vi "Init_Test.vi"(8 "error in (no error)":errorcluster caption="entrée d'erreur (pas d'erreur)", 11 "Get_Voltage en entrée":refnum<class "Start_Continuous_Ana.lvclass">) -> (0 "error out":errorcluster caption="sortie d'erreur", 3 "Get_Voltage en sortie":refnum<class "Start_Continuous_Ana.lvclass">)   [LabVIEW 2020, in "Library Test.lvlib" / "Start_Continuous_Ana.lvclass"]
uses:
  Start_Continuous_Ana.lvclass
  C:/Users/ngarcin/OneDrive - Altyor/Standard TB/Suite TB45/Class/Test/Test (Default)/Test (Default).lvclass
  Commun VI/TypeDef/Commande Test/Commande Value Type.ctl
  Commun VI/TypeDef/Commande Test/Commande Type Test.ctl
  Commun VI/TypeDef/Variable Printable.ctl
  Test_Wtih_Instr/Test_With_Inst.lvclass
  Instrument/Instrument (Default)/Class Instrument (Default).lvclass
  Commun VI/Library Commun.lvlib
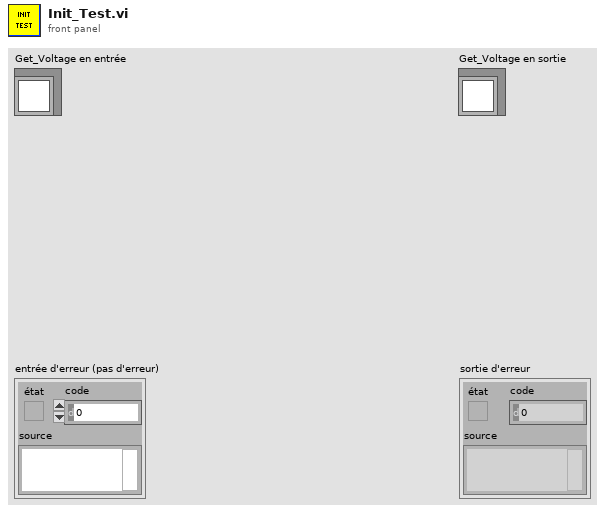
[diagram p1: front panel]
types:
  T1 = typedef "Variable Printable.ctl" = string
  T2 = enum16{"Get Variable", "Get All Variables", "Set Variable", "Delete Variable", "Delete All Variable"}
  T3 = typedef "Library Commun.lvlib/Commande Type Test.ctl" = enum16{"Function", "Test", "Calculation"}
  T4 = typedef "Library Commun.lvlib/Commande Value Type.ctl" = enum16{"None", "String", "Number", "Timestamp", "Boolean", "Array"}
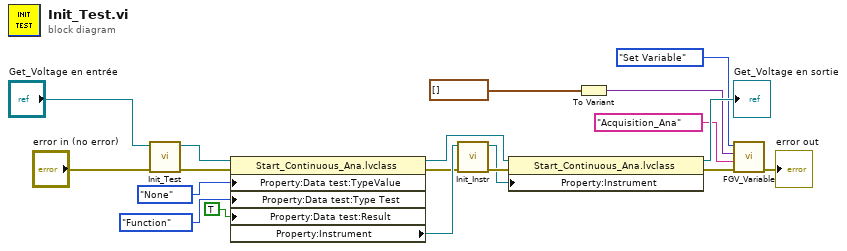
[diagram p0: block diagram]
diagram:
  n1 = call-parent "Init_Test.vi"("error in (no error)"="error in (no error)", "Test_With_Inst en entrée"="Get_Voltage en entrée") -> ("error out"=w16:errorcluster, "Test_With_Inst en sortie"=w17:refnum<class "Start_Continuous_Ana.lvclass">)  [unwired: 8 in]
  n2 = property class="Start_Continuous_Ana.lvclass"(reference=w17, error in=w16, "Property:Data test:TypeValue"=Commande_Value_Type."None" ("TypeValue"), "Property:Data test:Type Test"=Commande_Type_Test."Function" ("Type Test"), "Property:Data test:Result"=TRUE ("Result")) -> (reference out=w11:refnum<class "Start_Continuous_Ana.lvclass">, error out=w1:errorcluster, "Property:Instrument"=w2:refnum<class "Class Instrument (Default).lvclass">)
  n3 = call-dynamic "Init_Instr.vi"("error in (no error)"=w1, "Class Instrument (Default) en entrée"=w2) -> ("error out"=w12:errorcluster, "Class Instrument (Default) en sortie"=w10:refnum<class "Class Instrument (Default).lvclass">)  [unwired: 8 in]
  n4 = property class="Start_Continuous_Ana.lvclass"(reference=w11, error in=w12, "Property:Instrument"=w10) -> (reference out=→"Get_Voltage en sortie":refnum<class "Start_Continuous_Ana.lvclass">, error out=w4:errorcluster)
  n5 = To Variant(anything=waveform(dbl)[] [] ("data")) -> (Variant=w8:variant)
  n6 = call "FGV_Variable.vi"("error in (no error)"=w4, "Variable"=T1 "Acquisition_Ana", "Data In"=w8, "Function"=T2."Set Variable") -> ("error out"=→"error out":errorcluster)  [unwired: 5 in, 2 out]
